vi "auto tether saver.vi"(9 "Current Location":T1 {"Position"."Position Y" format="%#.3f"; "Position"."Position X" format="%#.3f"}, 10 "TraceName":string, 11 "List of devices":T2 {"List of locations"."Position"."Position Y" format="%#.3f"; "List of locations"."Position"."Position X" format="%#.3f"}) -> (0 "Found?":bool, 1 "Location of input":T1 {"Position"."Position Y" format="%#.3f"; "Position"."Position X" format="%#.3f"}, 3 "List of devices 2":T2 {"List of locations"."Position"."Position Y" format="%#.3f"; "List of locations"."Position"."Position X" format="%#.3f"})   [LabVIEW 2017]
uses:
  device_list.ctl
  device.ctl
  location.ctl
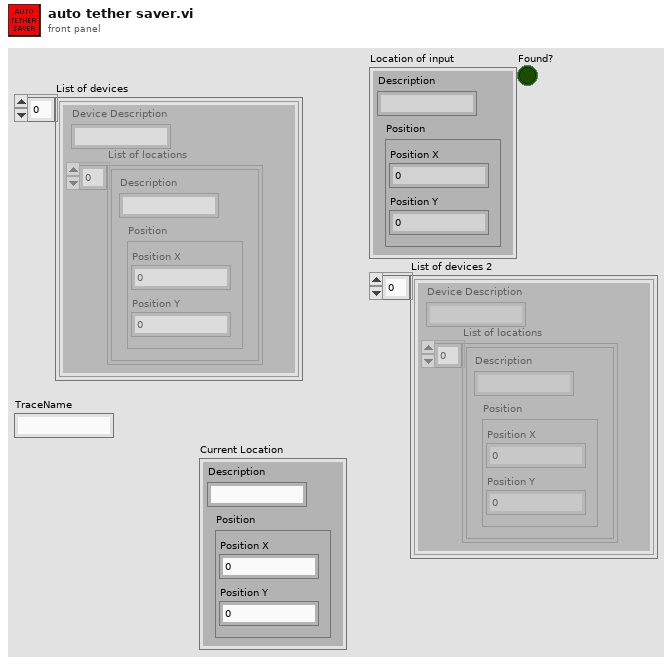
[diagram p1: front panel]
types:
  T1 = typedef "location.ctl" = cluster{"Description":string, "Position":cluster{"Position X":dbl, "Position Y":dbl}}
  T2 = typedef "device_list.ctl" = T3[]
  T3 = typedef "device.ctl" = cluster{"List of locations":T1[], "Device Description":string}
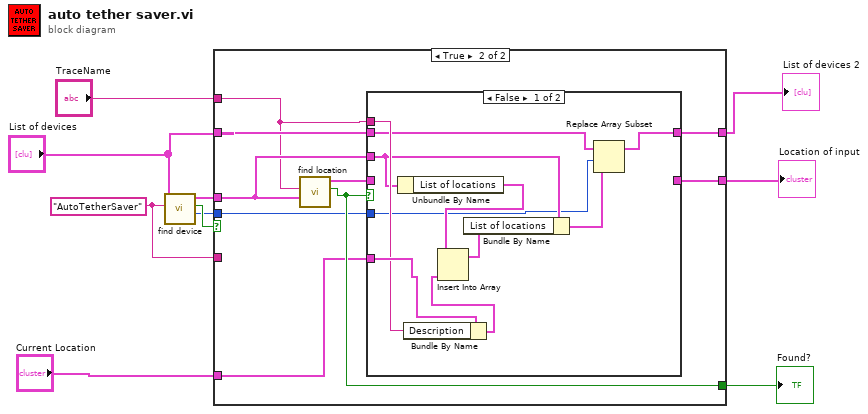
[diagram p0: block diagram]
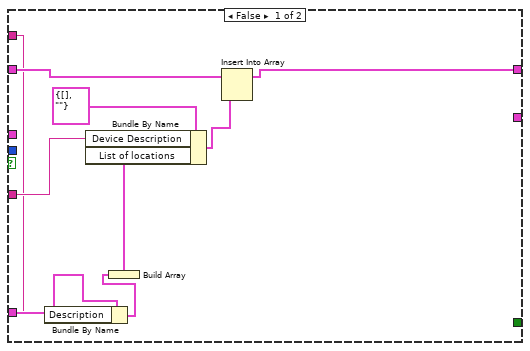
[diagram p2: hidden frame]
diagram:
  w3 = "AutoTetherSaver" ("Device Description")
  n1 = call "find device.vi"("Device Description"=w3, "List of devices"="List of devices") -> ("Index of device"=w1:i32, "Found?"=w9:bool, "Defualt Device"=w10:T3)  [unwired: 7 in]
  n2 = case shown="True" w9 {
    tunnel: w10 -> [_ w23]
    tunnel: "TraceName" -> [w12 w21]
    tunnel: [_ w27] -> w7
    tunnel: [_ w26] -> w6
    tunnel: "List of devices" -> [w19 w25]
    tunnel: [w15 w24] -> w4
    tunnel: w3 -> [w17 _]
    tunnel: "Current Location" -> [w13 w22]
    tunnel: w1 -> [_ w20]
    frame False {
      n3 = Bundle By Name(cluster=w13, "Description"=w12) -> (w11:T1)
      n4 = Build Array(w11) -> (w14:T1[])
      n5 = Bundle By Name(cluster=T3 {"List of locations"=[], "Device Description"=""} ("new element/subarray"), "Device Description"=w17, "List of locations"=w14) -> (w16:T3)
      n6 = Insert Into Array(array=w19, new element=w16) -> (w15:T2)  [unwired: 1 in]
    }
    frame True {
      n7 = call "find location.vi"("Location Description"=w21, "Defualt Device"=w23) -> ("Found?"=w26:bool, "Location of input"=w28:T1)  [unwired: 7 in, 1 out]
      n8 = case shown="False" w26 {
        tunnel: w28 -> [_ w40]
        tunnel: [_ w40] -> w27
        tunnel: w25 -> [w33 w39]
        tunnel: [w30 w39] -> w24
        tunnel: w23 -> [w32 _]
        tunnel: w22 -> [w36 _]
        tunnel: w21 -> [w35 _]
        tunnel: w20 -> [w31 _]
        frame False {
          n9 = Unbundle By Name(w32) -> ("List of locations"=w38:T1[])
          n10 = Bundle By Name(cluster=w36, "Description"=w35) -> (w34:T1)
          n11 = Insert Into Array(array=w38, new element=w34) -> (w37:T1[])  [unwired: 1 in]
          n12 = Bundle By Name(cluster=w32, "List of locations"=w37) -> (w29:T3)
          n13 = Replace Array Subset(array=w33, new element=w29, index=w31) -> (w30:T2)
        }
        frame True {
        }
      }
    }
  }
  "Location of input" <- w7
  "Found?" <- w6
  "List of devices 2" <- w4
